vi "FTW-Message-Initialize.vi"(0 "FTW Message":refnum<class "FTW-Message.lvclass">, 5 "Message":string, 11 "error in":errorcluster) -> (4 "FTW Message out":refnum<class "FTW-Message.lvclass">, 15 "error out":errorcluster)   [LabVIEW 2013, in "FTW-Actor.lvlib" / "FTW-Message.lvclass"]
uses:
  FTW-Message.lvclass
  FTW-Message.lvclass/FTW-Message.ctl
panel:
  # "Inputs"
  # "Outputs"
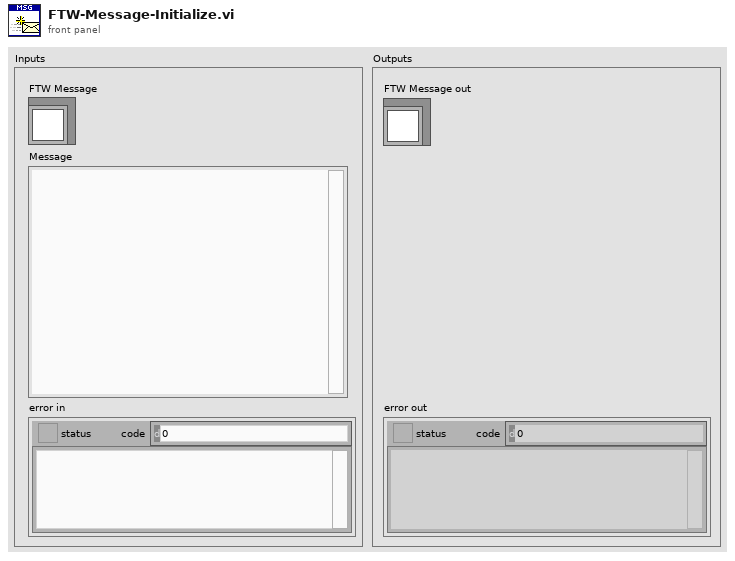
[diagram p1: front panel]
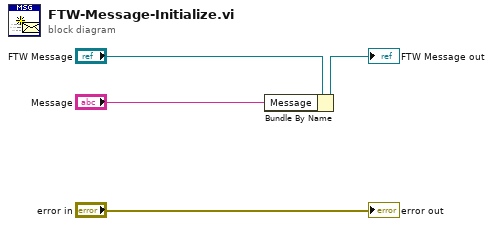
[diagram p0: block diagram]
diagram:
  n1 = Bundle By Name(cluster="FTW Message", "Message"="Message") -> (→"FTW Message out":refnum<class "FTW-Message.lvclass">)
  "error out" <- "error in"
